vi "fpga_Instantaneous Reset.vi"(6 "instantaneous reset after tripping? (F)":bool, 8 "input valid":bool=TRUE, 9 "dt/T":fxp<+/-,32,1>, 11 "previous integrated value":fxp<+,32,0>) -> (3 "instantaneous reset?":bool)   [LabVIEW 2012, in "NI_EP_Protection_FPGA.lvlib"]
uses:
  <vilib>/addons/Electrical Power/Protection/NI_EP_Protection_FPGA.lvlib
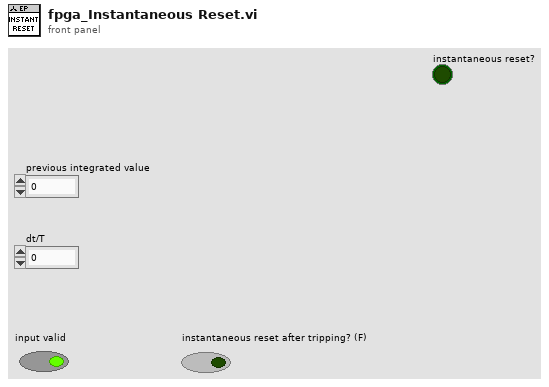
[diagram p1: front panel]
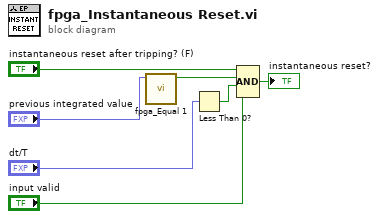
[diagram p0: block diagram]
diagram:
  n1 = call <vilib>:"fpga_Equal 1.vi"("data in 32.0"="previous integrated value") -> ("=1?"=w2:bool)  [unwired: 10 in]
  n2 = Less Than 0?(x="dt/T") -> (x < 0?=w7:bool)
  n3 = Compound Arithmetic op=AND("instantaneous reset after tripping? (F)", w2, w7, "input valid") -> (→"instantaneous reset?":bool)
